vi "Condition OpMap.vi"() -> (0 "OPERATORS":string)   [LabVIEW 2011]
uses:
  Condition Operators.ctl
  Fields/Field DataTypes.ctl
panel:
  in  "Condition Operators":T1
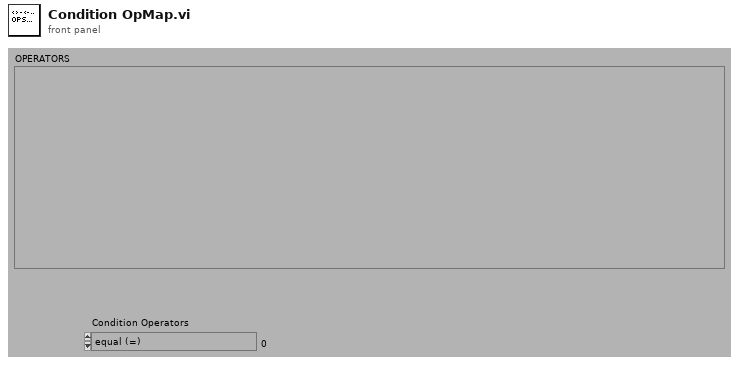
[diagram p1: front panel]
types:
  T1 = typedef "Condition Operators.ctl" = enum16{"equal (=)", "not equal (\\u2260)", "less than (<)", "less than or equal (\\u2264)", "greater than (>)", "greater than or equal (\\u2265)", "contains", "does not contain"}
  T2 = typedef "Field DataTypes.ctl" = enum32{"text", "numeric", "list", "timestamp", "boolean"}
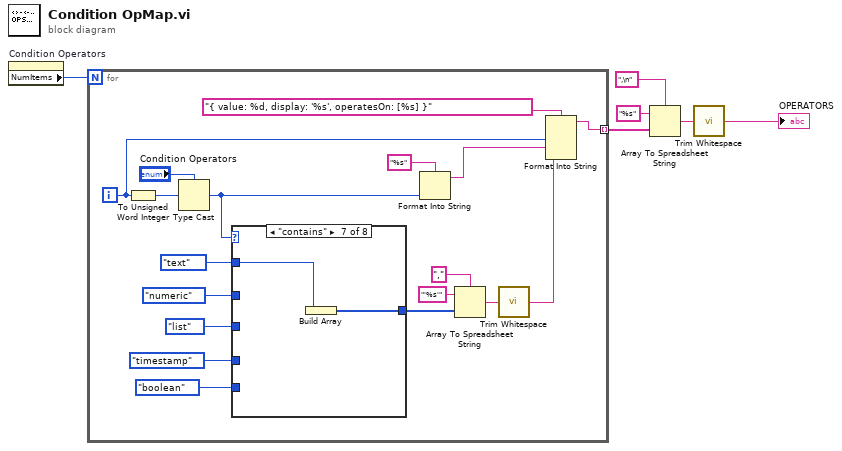
[diagram p0: block diagram]
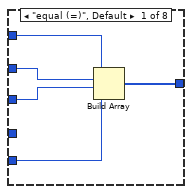
[diagram p2: hidden frame]
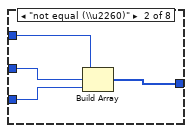
[diagram p3: hidden frame]
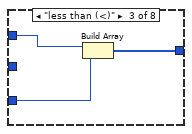
[diagram p4: hidden frame]
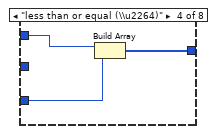
[diagram p5: hidden frame]
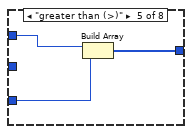
[diagram p6: hidden frame]
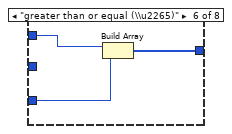
[diagram p7: hidden frame]
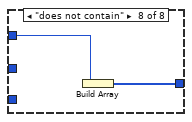
[diagram p8: hidden frame]
diagram:
  n1 = property on="Condition Operators" class="Enum (strict)"() -> ("NumItems"=w6:u32)  [unwired: 2 in, 2 out]
  n2 = for {
    N: w6 -> [_]
    tunnel: [w8] -> w4 mode=indexing
    i -> [w7]
    n3 = To Unsigned Word Integer(number=w7) -> (unsigned 16bit integer=w19:u16)
    n4 = Type Cast(type="Condition Operators", x=w19) -> (*(type *) &x=w12:T1)
    n5 = case shown="\"contains\"" w12 {
      tunnel: Field_DataTypes."text" ("Field DataType") -> [w29 w33 _ _ _ _ w46 w48]
      tunnel: Field_DataTypes."numeric" ("Field DataType") -> [w28 w32 w36 w39 w42 w45 _ _]
      tunnel: Field_DataTypes."list" ("Field DataType") -> [w27 w31 _ _ _ _ _ _]
      tunnel: Field_DataTypes."timestamp" ("Field DataType") -> [_ _ w35 w38 w41 w44 _ _]
      tunnel: [w26 w30 w34 w37 w40 w43 w47 w49] -> w15
      tunnel: Field_DataTypes."boolean" ("Field DataType") -> [w25 _ _ _ _ _ _ _]
      frame "equal (=)", Default {
        n6 = Build Array(w29, w28, w27, w25) -> (w26:T2[])
      }
      frame "not equal (\\u2260)" {
        n7 = Build Array(w33, w32, w31) -> (w30:T2[])
      }
      frame "less than (<)" {
        n8 = Build Array(w36, w35) -> (w34:T2[])
      }
      frame "less than or equal (\\u2264)" {
        n9 = Build Array(w39, w38) -> (w37:T2[])
      }
      frame "greater than (>)" {
        n10 = Build Array(w42, w41) -> (w40:T2[])
      }
      frame "greater than or equal (\\u2265)" {
        n11 = Build Array(w45, w44) -> (w43:T2[])
      }
      frame "contains" {
        n12 = Build Array(w46) -> (w47:T2[])
      }
      frame "does not contain" {
        n13 = Build Array(w48) -> (w49:T2[])
      }
    }
    n14 = Format Into String(format string="%s", w12) -> (resulting string=w10:string)  [unwired: 2 in, 1 out]
    n15 = Array To Spreadsheet String(delimiter (Tab)=",", array=w15, 3:"'%s'") -> (spreadsheet string=w18:string)
    n16 = call <vilib>:"Trim Whitespace.vi"("string"=w18) -> ("trimmed string"=w13:string)  [unwired: 1 in]
    n17 = Format Into String(format string="{ value: %d, display: '%s', operatesOn: [%s] }", w7, w10, w13) -> (resulting string=w8:string)  [unwired: 2 in, 1 out]
  }
  n18 = Array To Spreadsheet String(delimiter (Tab)=",\n", array=w4, 3:"%s" ("format string")) -> (spreadsheet string=w5:string)
  n19 = call <vilib>:"Trim Whitespace.vi"("string"=w5) -> ("trimmed string"=→"OPERATORS":string)  [unwired: 1 in]
